vi "IO_DataQCommandwRetry.vi"(8 "error in (no error)":errorcluster, 10 "Command":string="stop", 11 "VISA Refnum in":refnum<visa-resource-name>) -> (0 "error out":errorcluster, 1 "read buffer":string, 3 "VISA Refnum out":refnum<visa-resource-name>)   [LabVIEW 2024]
uses:
  <vilib>/regexp/Match Regular Expression.xnode
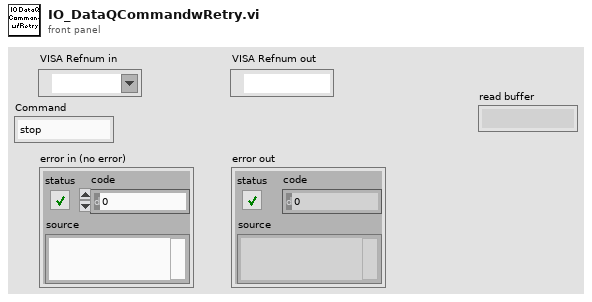
[diagram p1: front panel]
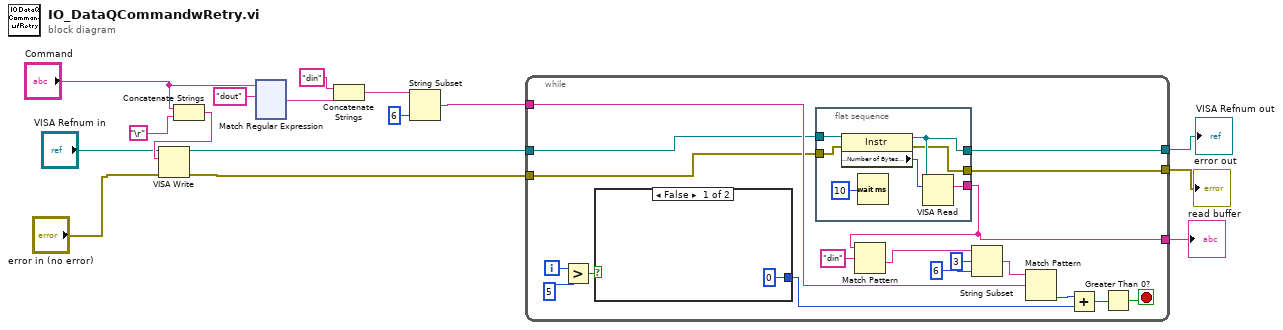
[diagram p0: block diagram]
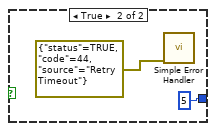
[diagram p2: hidden frame]
diagram:
  n1 = Concatenate Strings("Command", "\r") -> (w13:string)
  n2 = VISA Write(VISA resource name="VISA Refnum in", write buffer=w13, error in (no error)="error in (no error)") -> (VISA resource name out=w10:refnum<visa-resource-name>, error out=w11:errorcluster)  [unwired: 1 out]
  n3 = xnode "Match Regular Expression"("input string"="Command", "regular expression"="dout") -> ("after match"=w4:string)  [unwired: 4 in, 4 out]
  n4 = Concatenate Strings("din" ("string"), w4) -> (w3:string)
  n5 = String Subset(string=w3, length (rest)=6 ("length (rest)")) -> (substring=w1:string)  [unwired: 1 in]
  n6 = while {
    tunnel: [w27] -> w15
    tunnel: [w26] -> w16
    tunnel: w1 -> [w25]
    tunnel: [w20] -> w14
    tunnel: w11 -> [w24]
    tunnel: w10 -> [w23]
    i -> [w34]
    stop <- w29 stop-if-true
    n7 = Greater?(x=w34, y=5) -> (0:w32:bool)
    n8 = case shown="False" w32 {
      tunnel: [0 5] -> w28
      frame False {
      }
      frame True {
        n9 = call <vilib>:"Simple Error Handler.vi"("error in (no error)"=errorcluster {"status"=TRUE, "code"=44, "source"="Retry Timeout"} ("error out")) -> ()  [unwired: 4 in, 5 out]
      }
    }
    n10 = flat-sequence {
      tunnel: [w42] -> w20
      tunnel: [w41] -> w27
      tunnel: [w40] -> w26
      tunnel: w24 -> [w39]
      tunnel: w23 -> [w38]
      frame #0 {
        n11 = property class="Instr"(reference=w38, error in=w39) -> (reference out=w41:refnum<visa-resource-name>, error out=w40:errorcluster, "Serial Settings:Number of Bytes at Serial Port"=w43:u32)
        n12 = Wait (ms)(milliseconds to wait=u32 10) -> ()  [unwired: 1 out]
        n13 = VISA Read(VISA resource name=w41, byte count=w43) -> (read buffer=w42:string)  [unwired: 1 in, 3 out]
      }
    }
    n14 = Match Pattern(string=w20, regular expression="din") -> (after substring=w18:string)  [unwired: 1 in, 3 out]
    n15 = String Subset(string=w18, offset (0)=3, length (rest)=6 ("length (rest)")) -> (substring=w21:string)
    n16 = Match Pattern(string=w21, regular expression=w25) -> (offset past match=w31:i32)  [unwired: 1 in, 3 out]
    n17 = Add(x=w31, y=w28) -> (x+y=w30:i32)
    n18 = Greater Than 0?(x=w30) -> (x > 0?=w29:bool)
  }
  "error out" <- w16
  "VISA Refnum out" <- w15
  "read buffer" <- w14
